vi "BuildTestFromProjectItem.vi"(8 "error in (no error)":errorcluster, 10 "ProjectItem Refnum":refnum<vi>, 11 "LVUnitTestBuilder in":refnum<class "LVUnitTestBuilder.lvclass">) -> (0 "error out":errorcluster, 2 "Test":refnum<class "Test.lvclass">, 3 "LVUnitTestBuilder out":refnum<class "LVUnitTestBuilder.lvclass">)   [LabVIEW 2017, in "LVUnitTestBuilder.lvclass"]
doc: "Builds a test from the specified <B>ProjectItem</B>."
uses:
  LVUnitTestBuilder.lvclass
  Test/Test.lvclass
  <vilib>/Utility/error.llb/Error Cluster From Error Code.vi
  <vilib>/ErrorRing/Error Ring.xnode
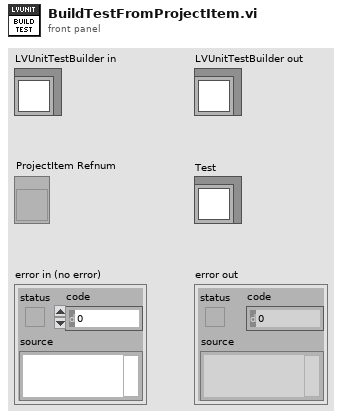
[diagram p1: front panel]
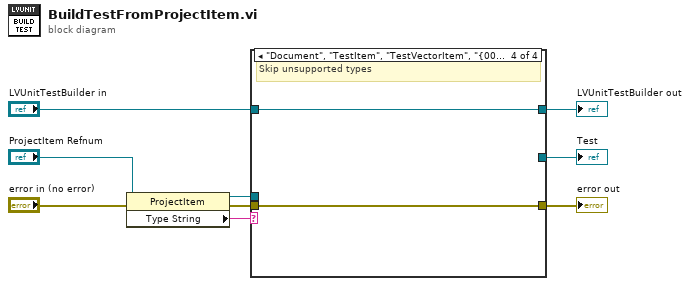
[diagram p0: block diagram]
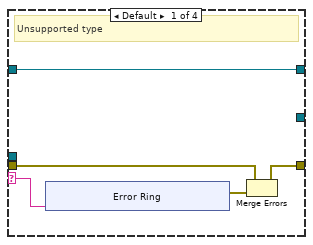
[diagram p2: hidden frame]
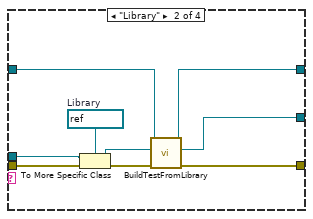
[diagram p3: hidden frame]
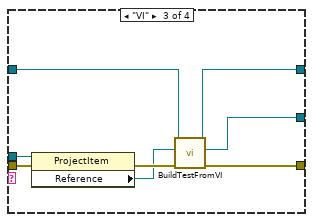
[diagram p4: hidden frame]
diagram:
  n1 = property class="ProjectItem"(reference="ProjectItem Refnum", error in="error in (no error)") -> (reference out=w2:refnum<vi>, error out=w6:errorcluster, "Type String"=w8:string)
  n2 = case shown="\"Document\", \"TestItem\", \"TestVectorItem\", \"{00000000-0000-0000-0000-000000000000}\"" w8 {
    selector: w8 -> [w13 _ _ _]
    tunnel: [w10 w29 w38 w39] -> w7
    tunnel: w6 -> [w12 w30 w34 w39]
    tunnel: "LVUnitTestBuilder in" -> [w14 w28 w37 w40]
    tunnel: [w14 w27 w36 w40] -> w4
    tunnel: [_ w26 w35 _] -> w3
    tunnel: w2 -> [_ w23 w32 _]
    frame Default {
      # "Unsupported type"
      n3 = xnode "Error Ring"("parameter 0"=w13) -> ("error out"=w11:errorcluster)
      n4 = Merge Errors(w12, w11) -> (w10:errorcluster)
    }
    frame "Library" {
      w22 = refnum<vi> refnum  # Library
      n5 = To More Specific Class(target class=w22, reference=w23, error in=w30) -> (specific class reference=w24:refnum<vi>, error out=w25:errorcluster)
      n6 = call "BuildTestFromLibrary.vi"("error in (no error)"=w25, "Library Refnum"=w24, "LVUnitTestBuilder in"=w28) -> ("error out"=w29:errorcluster, "Test"=w26:refnum<class "Test.lvclass">, "LVUnitTestBuilder out"=w27:refnum<class "LVUnitTestBuilder.lvclass">)  [unwired: 6 in]
    }
    frame "VI" {
      n7 = property class="ProjectItem"(reference=w32, error in=w34) -> (error out=w33:errorcluster, "Reference"=w31:refnum<vi>)  [unwired: 1 out]
      n8 = call "BuildTestFromVI.vi"("error in (no error)"=w33, "VI Refnum"=w31, "LVUnitTestBuilder in"=w37) -> ("error out"=w38:errorcluster, "Test"=w35:refnum<class "Test.lvclass">, "LVUnitTestBuilder out"=w36:refnum<class "LVUnitTestBuilder.lvclass">)  [unwired: 6 in]
    }
    frame "Document", "TestItem", "TestVectorItem", "{00000000-0000-0000-0000-000000000000}" {
      # "Skip unsupported types"
    }
  }
  "error out" <- w7
  "LVUnitTestBuilder out" <- w4
  "Test" <- w3
